vi "正逆解随机测试.vi"() -> ()   [LabVIEW 2015]
uses:
  <vilib>/Utility/file.llb/Write To Spreadsheet File (DBL).vi
panel:
  out "误差2":dbl[](array[numeric])
  out "验证输出 2":dbl[](array[numeric])=[-2177.0, -1.4612052517330483e-10, 558.0000000005964, 1.0] format="%#.6f"
  out "运动学逆解2":dbl[](array[numeric])
  in  "随机测试次数":dbl
  out "angle6":dbl
  out "angle5":dbl
  out "angle4":dbl
  out "angle3":dbl
  out "angle2":dbl
  out "angle1":dbl
  out "误差":dbl[](array[numeric])
  out "逆运动学输出":dbl[](array[numeric])=[0.0, 0.0, 0.0, 0.0, 4.859887553275934e-12, 0.0] format="%#.3f"
  out "正解输出":dbl[](array[numeric])=[0.19999999999996898, -1.0341155355512858e-14, 0.3000000000000207] format="%#.6f"
  out "验证输出":dbl[](array[numeric])=[0.19999999999996898, -1.0341155355512858e-14, 0.3000000000000207] format="%#.6f"
  in  "关节数":dbl=6.0
  in  "正运动学输入":dbl[](array[numeric])=[0.0, 0.0, 0.0, 0.0, 0.0, 0.0]
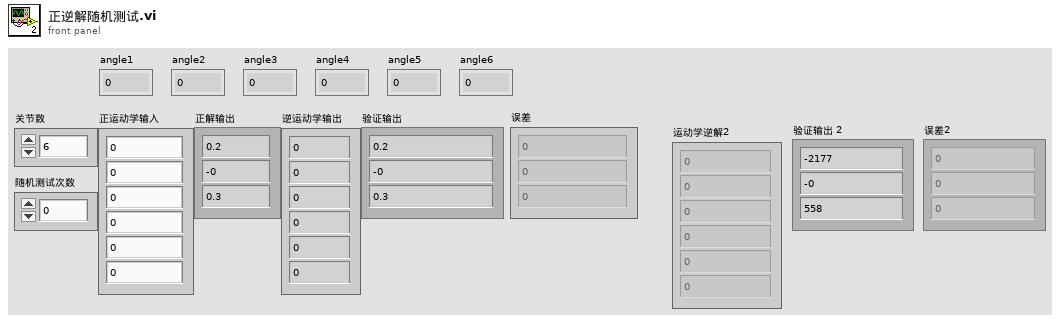
[diagram p1: front panel]
types:
  T1 = typedef "Real Matrix NI_Silver.ctl" = dbl[][]
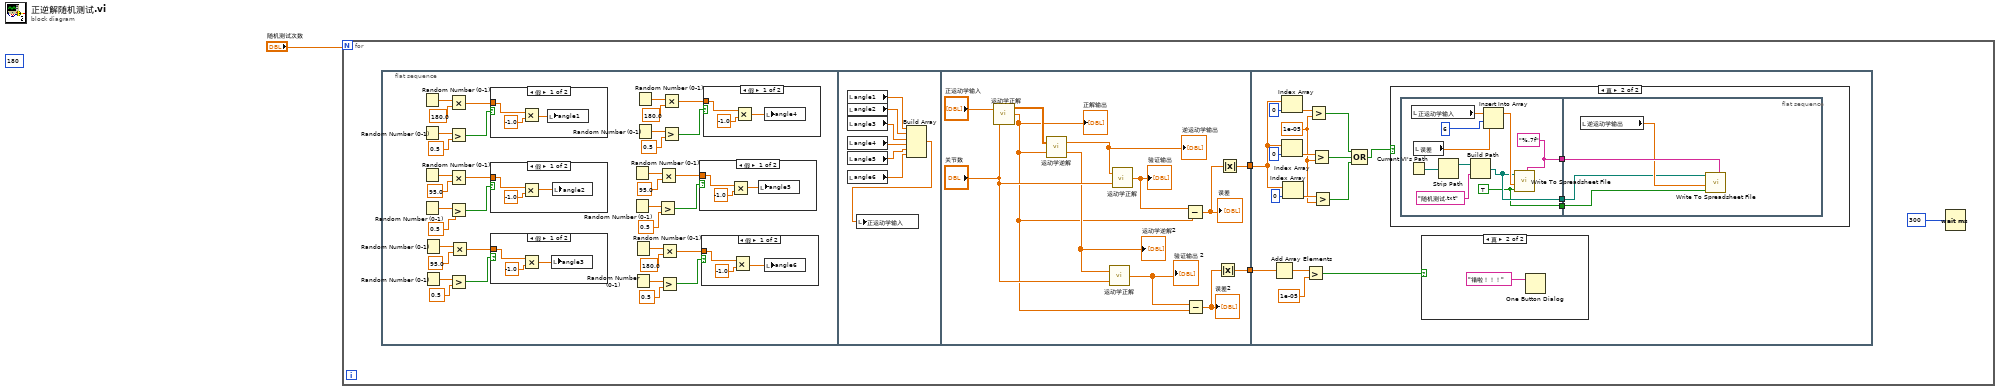
[diagram p0: block diagram]
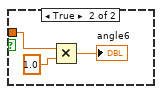
[diagram p2: hidden frame]
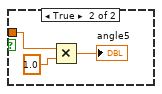
[diagram p3: hidden frame]
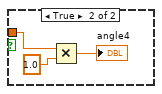
[diagram p4: hidden frame]
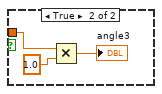
[diagram p5: hidden frame]
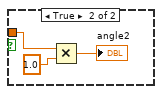
[diagram p6: hidden frame]
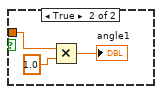
[diagram p7: hidden frame]
diagram:
  (unwired) 180
  n1 = for {
    N: "随机测试次数" -> [_]
    n2 = flat-sequence {
      tunnel: [w92] -> w4
      tunnel: [w84] -> w3
      tunnel: w4 -> [w108]
      tunnel: w3 -> [w99]
      frame #0 {
        n3 = Random Number (0-1)() -> (number: 0 to 1=w40:dbl)
        n4 = Random Number (0-1)() -> (number: 0 to 1=w38:dbl)
        n5 = Random Number (0-1)() -> (number: 0 to 1=w34:dbl)
        n6 = Random Number (0-1)() -> (number: 0 to 1=w32:dbl)
        n7 = Random Number (0-1)() -> (number: 0 to 1=w28:dbl)
        n8 = Random Number (0-1)() -> (number: 0 to 1=w26:dbl)
        n9 = Greater?(x=w38, y=0.5) -> (0:w36:bool)
        n10 = Greater?(x=w32, y=0.5) -> (0:w30:bool)
        n11 = Multiply(x=w40, y=180.0) -> (x*y=w35:dbl)
        n12 = Multiply(x=w34, y=95.0) -> (x*y=w29:dbl)
        n13 = Greater?(x=w26, y=0.5) -> (0:w24:bool)
        n14 = Multiply(x=w28, y=95.0) -> (x*y=w23:dbl)
        n15 = case shown="假" w36 {
          tunnel: w35 -> [w73 w76]
          frame False {
            n16 = Multiply(x=w73, y=-1.0) -> (x*y=w71:dbl)
            n17 = local write "angle1"(w71) -> ()
          }
          frame True {
            n18 = Multiply(x=w76, y=1.0) -> (x*y=→"angle1":dbl)
          }
        }
        n19 = case shown="假" w30 {
          tunnel: w29 -> [w67 w70]
          frame False {
            n20 = Multiply(x=w67, y=-1.0) -> (x*y=w65:dbl)
            n21 = local write "angle2"(w65) -> ()
          }
          frame True {
            n22 = Multiply(x=w70, y=1.0) -> (x*y=→"angle2":dbl)
          }
        }
        n23 = case shown="假" w24 {
          tunnel: w23 -> [w61 w64]
          frame False {
            n24 = Multiply(x=w61, y=-1.0) -> (x*y=w59:dbl)
            n25 = local write "angle3"(w59) -> ()
          }
          frame True {
            n26 = Multiply(x=w64, y=1.0) -> (x*y=→"angle3":dbl)
          }
        }
        n27 = Random Number (0-1)() -> (number: 0 to 1=w16:dbl)
        n28 = Random Number (0-1)() -> (number: 0 to 1=w14:dbl)
        n29 = Random Number (0-1)() -> (number: 0 to 1=w10:dbl)
        n30 = Random Number (0-1)() -> (number: 0 to 1=w8:dbl)
        n31 = Random Number (0-1)() -> (number: 0 to 1=w22:dbl)
        n32 = Random Number (0-1)() -> (number: 0 to 1=w20:dbl)
        n33 = Greater?(x=w14, y=0.5) -> (0:w12:bool)
        n34 = Multiply(x=w16, y=95.0) -> (x*y=w11:dbl)
        n35 = Greater?(x=w8, y=0.5) -> (0:w6:bool)
        n36 = Multiply(x=w10, y=180.0) -> (x*y=w5:dbl)
        n37 = Greater?(x=w20, y=0.5) -> (0:w18:bool)
        n38 = Multiply(x=w22, y=180.0) -> (x*y=w17:dbl)
        n39 = case shown="假" w12 {
          tunnel: w11 -> [w49 w52]
          frame False {
            n40 = Multiply(x=w49, y=-1.0) -> (x*y=w47:dbl)
            n41 = local write "angle5"(w47) -> ()
          }
          frame True {
            n42 = Multiply(x=w52, y=1.0) -> (x*y=→"angle5":dbl)
          }
        }
        n43 = case shown="假" w6 {
          tunnel: w5 -> [w43 w46]
          frame False {
            n44 = Multiply(x=w43, y=-1.0) -> (x*y=w41:dbl)
            n45 = local write "angle6"(w41) -> ()
          }
          frame True {
            n46 = Multiply(x=w46, y=1.0) -> (x*y=→"angle6":dbl)
          }
        }
        n47 = case shown="假" w18 {
          tunnel: w17 -> [w55 w58]
          frame False {
            n48 = Multiply(x=w55, y=-1.0) -> (x*y=w53:dbl)
            n49 = local write "angle4"(w53) -> ()
          }
          frame True {
            n50 = Multiply(x=w58, y=1.0) -> (x*y=→"angle4":dbl)
          }
        }
      }
      frame #1 {
        n51 = local read "angle1"() -> (w83:dbl)
        n52 = local read "angle2"() -> (w82:dbl)
        n53 = local read "angle3"() -> (w81:dbl)
        n54 = local read "angle4"() -> (w80:dbl)
        n55 = local read "angle5"() -> (w79:dbl)
        n56 = local read "angle6"() -> (w78:dbl)
        n57 = Build Array(w83, w82, w81, w80, w79, w78) -> (w77:dbl[])
        n58 = local write "正运动学输入"(w77) -> ()
      }
      frame #2 {
        n59 = call "运动学正解.vi"("正运动学输入"="正运动学输入", "关节数"="关节数") -> ("Tx"=w94:T1, "正解输出"=w86:dbl[])  [unwired: 1 out]
        "正解输出" <- w86
        n60 = call "运动学逆解.vi"("逆运动学输入"=w86, "机械臂末端姿态"=w94) -> ("运动学逆解2"=w88:dbl[], "运动学逆解1"=w90:dbl[])
        "逆运动学输出" <- w90
        "运动学逆解2" <- w88
        n61 = call "运动学正解.vi"("正运动学输入"=w88, "关节数"="关节数") -> ("正解输出"=w87:dbl[])  [unwired: 2 out]
        "验证输出 2" <- w87
        n62 = call "运动学正解.vi"("正运动学输入"=w90, "关节数"="关节数") -> ("正解输出"=w93:dbl[])  [unwired: 2 out]
        "验证输出" <- w93
        n63 = Subtract(x=w93, y=w86) -> (x-y=w91:dbl[])
        "误差" <- w91
        n64 = Subtract(x=w87, y=w86) -> (x-y=w85:dbl[])
        "误差2" <- w85
        n65 = Absolute Value(x=w85) -> (abs(x)=w84:dbl[])
        n66 = Absolute Value(x=w91) -> (abs(x)=w92:dbl[])
      }
      frame #3 {
        w104 = 1e-05
        n67 = Add Array Elements(numeric array=w99) -> (sum=w98:dbl)
        n68 = Index Array(array=w108, index=0) -> (element=w107:dbl)
        n69 = Index Array(array=w108, index=0) -> (element=w106:dbl)
        n70 = Index Array(array=w108, index=0) -> (element=w105:dbl)
        n71 = Greater?(x=w98, y=1e-05) -> (0:w96:bool)
        n72 = Greater?(x=w107, y=w104) -> (0:w103:bool)
        n73 = Greater?(x=w106, y=w104) -> (0:w102:bool)
        n74 = Greater?(x=w105, y=w104) -> (0:w101:bool)
        n75 = Compound Arithmetic op=OR(w103, w102, w101) -> (w100:bool)
        n76 = case shown="真" w100 {
          frame False {
          }
          frame True {
            n77 = flat-sequence {
              tunnel: [w118] -> w115
              tunnel: [w117] -> w114
              tunnel: [w116] -> w113
              tunnel: w115 -> [w129]
              tunnel: w114 -> [w127]
              tunnel: w113 -> [w126]
              frame #0 {
                w118 = "%.7f"
                w116 = TRUE
                n78 = Current VI's Path() -> (path=w121:path)
                n79 = local read "正运动学输入"() -> (w125:dbl[])
                n80 = local read "误差"() -> (w122:dbl[])
                n81 = Strip Path(path=w121) -> (stripped path=w120:path)  [unwired: 1 out]
                n82 = Build Path(base path=w120, name or relative path="随机测试.txt") -> (appended path=w117:path)
                n83 = Insert Into Array(array=w125, index=6, new element=w122) -> (w123:dbl[])
                n84 = call-poly <vilib>:"Write To Spreadsheet File.vi"("format (%.3f)"=w118, "append to file? (new file:F)"=w116, "1D data"=w123, "file path (dialog if empty)"=w117) -> ()  [unwired: 4 in, 1 out]
              }
              frame #1 {
                n85 = local read "逆运动学输出"() -> (w128:dbl[])
                n86 = call-poly <vilib>:"Write To Spreadsheet File.vi"("format (%.3f)"=w129, "append to file? (new file:F)"=w126, "1D data"=w128, "file path (dialog if empty)"=w127) -> ()  [unwired: 4 in, 1 out]
              }
            }
          }
        }
        n87 = case shown="真" w96 {
          frame False {
          }
          frame True {
            n88 = One Button Dialog(message="错啦！！！") -> ()  [unwired: 1 in, 1 out]
          }
        }
      }
    }
    n89 = Wait (ms)(milliseconds to wait=300) -> ()  [unwired: 1 out]
  }
